vi "[SubV]PEMG_Torque.vi"(4 "Assist?":bool=TRUE, 5 "GP Info":dbl[](array[numeric]), 6 "Max Assistance (Nm)":dbl format="%#_13g", 7 "L_Ext":dbl format="%#_13g", 8 "L_Flex":dbl format="%#_13g", 9 "R_Ext":dbl format="%#_13g", 10 "R_Flex":dbl format="%#_13g") -> (0 "L_torque":dbl format="%#_13g", 3 "R_torque":dbl format="%#_13g")   [LabVIEW 2018]
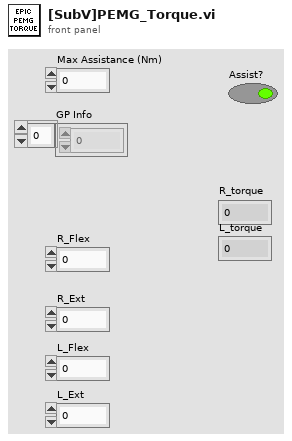
[diagram p1: front panel]
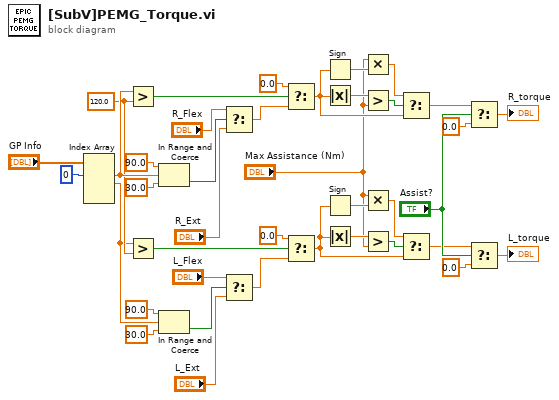
[diagram p0: block diagram]
diagram:
  w23 = 120.0 ("y")
  n1 = Index Array(array="GP Info", index #1=0 ("index")) -> (element #1=w29:dbl, element #2=w21:dbl)  [unwired: 3 in, 2 out]
  n2 = Greater?(x=w29, y=w23) -> (0:w26:bool)
  n3 = Greater?(x=w21, y=w23) -> (0:w24:bool)
  n4 = In Range and Coerce(upper limit=90.0, x=w29, lower limit=30.0) -> (In Range?=w35:bool)  [unwired: 1 out]
  n5 = In Range and Coerce(upper limit=90.0, x=w21, lower limit=30.0) -> (In Range?=w31:bool)  [unwired: 1 out]
  n6 = Select(t="R_Flex", s=w35, f="R_Ext") -> (s? t:f=w28:dbl)
  n7 = Select(t="L_Flex", s=w31, f="L_Ext") -> (s? t:f=w22:dbl)
  n8 = Select(t=0.0, s=w26, f=w28) -> (s? t:f=w16:dbl)
  n9 = Select(t=0.0, s=w24, f=w22) -> (s? t:f=w11:dbl)
  n10 = Sign(1:w16) -> (0:w18:dbl)
  n11 = Absolute Value(x=w16) -> (abs(x)=w20:dbl)
  n12 = Sign(1:w11) -> (0:w13:dbl)
  n13 = Absolute Value(x=w11) -> (abs(x)=w15:dbl)
  n14 = Multiply(x="Max Assistance (Nm)", y=w18) -> (x*y=w17:dbl)
  n15 = Greater?(x=w20, y="Max Assistance (Nm)") -> (0:w19:bool)
  n16 = Multiply(x="Max Assistance (Nm)", y=w13) -> (x*y=w12:dbl)
  n17 = Greater?(x=w15, y="Max Assistance (Nm)") -> (0:w14:bool)
  n18 = Select(t=w17, s=w19, f=w16) -> (s? t:f=w9:dbl)
  n19 = Select(t=w12, s=w14, f=w11) -> (s? t:f=w4:dbl)
  n20 = Select(t=w9, s="Assist?", f=0.0) -> (s? t:f=→"R_torque":dbl)
  n21 = Select(t=w4, s="Assist?", f=0.0) -> (s? t:f=→"L_torque":dbl)
